vi "CreateMeshgrid.vi"(11 "Cluster":T1) -> (2 "Y":dbl[][](array[numeric]), 3 "X":dbl[][](array[numeric]))   [LabVIEW 2015]
uses:
  <vilib>/gmath/interp.llb/Create Mesh Grid (2D) (x,y arrays).vi
  <vilib>/gmath/NI_Gmath.lvlib
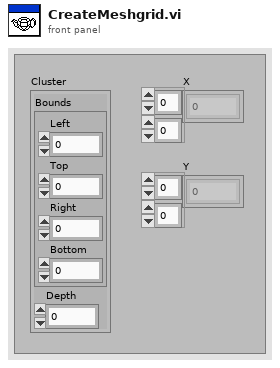
[diagram p1: front panel]
types:
  T1 = cluster{"Bounds":cluster{"Left":i16, "Top":i16, "Right":i16, "Bottom":i16}, "Depth":i16}
  T2 = cluster{"Bounds":cluster{"Left":i32, "Top":i32, "Right":i32, "Bottom":i32}, "Depth":i32}
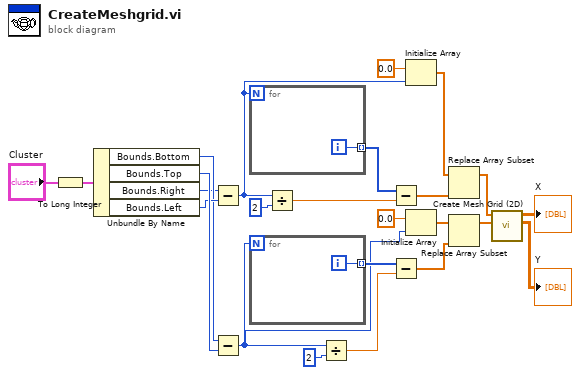
[diagram p0: block diagram]
diagram:
  n1 = To Long Integer(number="Cluster") -> (32bit integer=w5:T2)
  n2 = Unbundle By Name(w5) -> ("Bounds.Bottom"=w8:i32, "Bounds.Top"=w22:i32, "Bounds.Right"=w7:i32, "Bounds.Left"=w21:i32)
  n3 = Subtract(x=w7, y=w21) -> (x-y=w2:i32)
  n4 = Subtract(x=w8, y=w22) -> (x-y=w1:i32)
  n5 = for {
    N: w2 -> [_]
    tunnel: [w25] -> w17 mode=indexing
    i -> [w25]
  }
  n6 = for {
    N: w1 -> [_]
    tunnel: [w26] -> w16 mode=indexing
    i -> [w26]
  }
  n7 = Divide(x=w2, y=2) -> (x/y=w10:dbl)
  n8 = Divide(x=w1, y=2) -> (x/y=w13:dbl)
  n9 = Subtract(x=w17, y=w10) -> (x-y=w18:dbl[])
  n10 = Subtract(x=w16, y=w13) -> (x-y=w20:dbl[])
  n11 = Initialize Array(0.0, w2) -> (w4:dbl[])
  n12 = Initialize Array(0.0, w1) -> (w14:dbl[])
  n13 = Replace Array Subset(array=w4, new element=w18) -> (w19:dbl[])  [unwired: 1 in]
  n14 = Replace Array Subset(array=w14, new element=w20) -> (w15:dbl[])  [unwired: 1 in]
  n15 = call-poly <vilib>:"Create Mesh Grid (2D).vi"("y domain"=w15, "x domain"=w19) -> ("Y"=→"Y":dbl[][], "X"=→"X":dbl[][])  [unwired: 7 in, 1 out]
